vi "删除一维数组中0.vi"(11 "数组输入":u16[](array[numeric])) -> (3 "数组输出":u16[](array[numeric]))   [LabVIEW 2020]
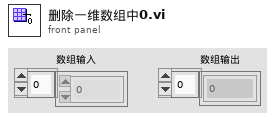
[diagram p1: front panel]
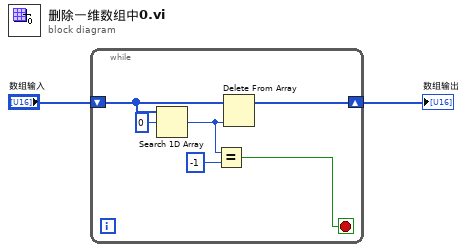
[diagram p0: block diagram]
diagram:
  n1 = while {
    shift-right: [w6] -> w2
    shift-left: "数组输入" -> [w7]
    stop <- w3 stop-if-true
    n2 = Search 1D Array(1D array=w7, element=u16 0 ("元素")) -> (index of element=w5:i32)  [unwired: 1 in]
    n3 = Equal?(x=w5, y=-1) -> (x = y?=w3:bool)
    n4 = Delete From Array(array=w7, index=w5) -> (array with subset deleted=w6:u16[])  [unwired: 1 in, 1 out]
  }
  "数组输出" <- w2
